vi "Modbus Data Massage New.vi"(10 "register values":u16[](array[numeric]), 11 "Cluster":T1) -> (2 "output cluster":cluster{"Control Name":string, "Value":dbl})   [LabVIEW 2020]
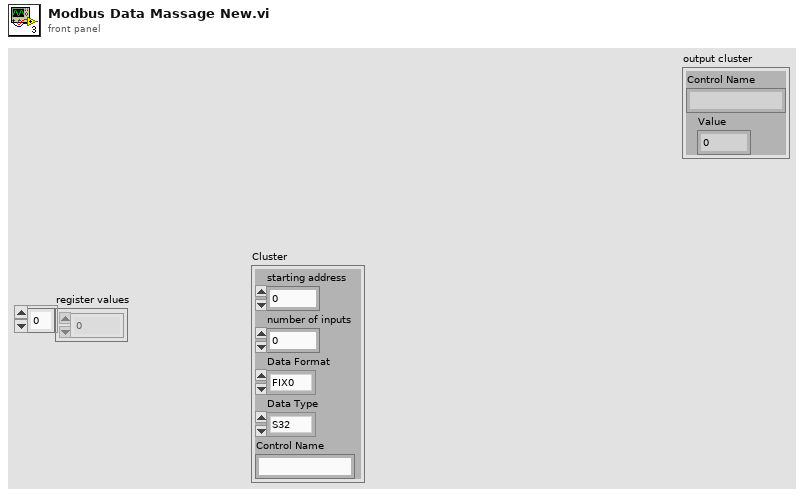
[diagram p1: front panel]
types:
  T1 = cluster{"starting address":u16, "number of inputs":u16, "Data Format":enum16{"FIX0", "FIX1", "FIX2", "FIX3", "FIX4", "FIX5", "FIX6"}, "Data Type":enum16{"S32", "U32", "U64", "S64"}, "Control Name":string}
  T2 = enum16{"FIX0", "FIX1", "FIX2", "FIX3", "FIX4", "FIX5", "FIX6"}
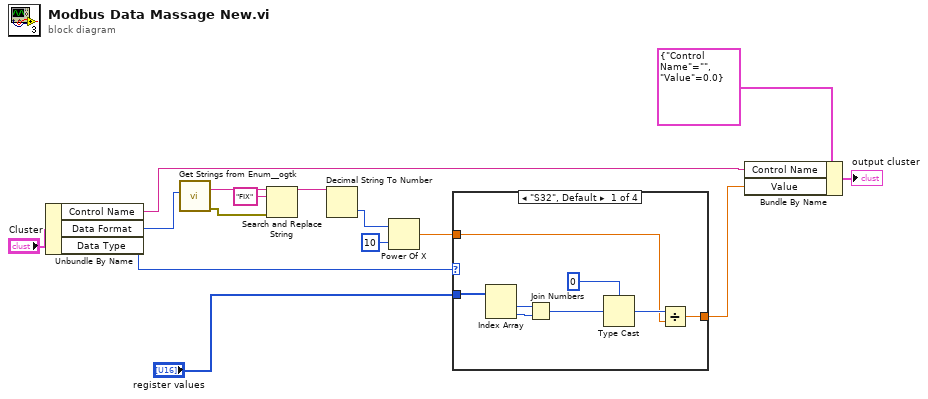
[diagram p0: block diagram]
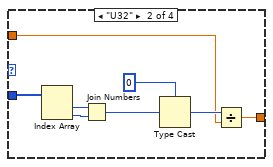
[diagram p2: hidden frame]
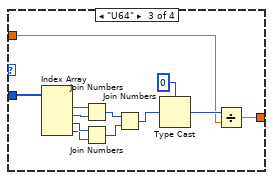
[diagram p3: hidden frame]
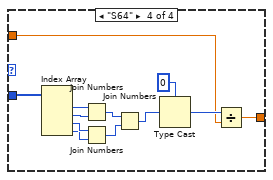
[diagram p4: hidden frame]
diagram:
  n1 = Unbundle By Name("Cluster") -> ("Control Name"=w3:string, "Data Format"=w6:T2, "Data Type"=w13:enum16{"S32", "U32", "U64", "S64"})
  n2 = call <userlib>:"Get Strings from Enum__ogtk.vi"("Enum"=w6) -> ("error out"=w12:errorcluster, "String Value"=w11:string)  [unwired: 7 in, 2 out]
  n3 = Search and Replace String(input string=w11, search string="FIX", error in=w12) -> (result string=w9:string)  [unwired: 5 in, 3 out]
  n4 = Decimal String To Number(string=w9) -> (number=w8:i32)  [unwired: 2 in, 1 out]
  n5 = Power Of X(1:10 ("x"), 2:w8) -> (0:w5:dbl)
  n6 = case shown="\"S32\", Default" w13 {
    tunnel: "register values" -> [w23 w31 w43 w55]
    tunnel: w5 -> [w17 w25 w38 w50]
    tunnel: [w16 w24 w37 w49] -> w2
    frame "S32", Default {
      n7 = Index Array(array=w23) -> (element #1=w22:u16, element #2=w21:u16)  [unwired: 2 in]
      n8 = Join Numbers(hi=w22, lo=w21) -> ((hi.lo)=w20:u32)
      n9 = Type Cast(type=0, x=w20) -> (*(type *) &x=w18:i32)
      n10 = Divide(x=w18, y=w17) -> (x/y=w16:dbl)
    }
    frame "U32" {
      n11 = Index Array(array=w31) -> (element #1=w30:u16, element #2=w29:u16)  [unwired: 2 in]
      n12 = Join Numbers(hi=w30, lo=w29) -> ((hi.lo)=w28:u32)
      n13 = Type Cast(type=u32 0, x=w28) -> (*(type *) &x=w26:u32)
      n14 = Divide(x=w26, y=w25) -> (x/y=w24:dbl)
    }
    frame "U64" {
      n15 = Index Array(array=w43) -> (element #1=w42:u16, element #2=w41:u16, element #3=w36:u16, element #4=w35:u16)  [unwired: 4 in]
      n16 = Join Numbers(hi=w42, lo=w41) -> ((hi.lo)=w34:u32)
      n17 = Join Numbers(hi=w36, lo=w35) -> ((hi.lo)=w33:u32)
      n18 = Join Numbers(hi=w34, lo=w33) -> ((hi.lo)=w32:u64)
      n19 = Type Cast(type=u64 0, x=w32) -> (*(type *) &x=w39:u64)
      n20 = Divide(x=w39, y=w38) -> (x/y=w37:dbl)
    }
    frame "S64" {
      n21 = Index Array(array=w55) -> (element #1=w54:u16, element #2=w53:u16, element #3=w48:u16, element #4=w47:u16)  [unwired: 4 in]
      n22 = Join Numbers(hi=w54, lo=w53) -> ((hi.lo)=w46:u32)
      n23 = Join Numbers(hi=w48, lo=w47) -> ((hi.lo)=w45:u32)
      n24 = Join Numbers(hi=w46, lo=w45) -> ((hi.lo)=w44:u64)
      n25 = Type Cast(type=i64 0, x=w44) -> (*(type *) &x=w51:i64)
      n26 = Divide(x=w51, y=w50) -> (x/y=w49:dbl)
    }
  }
  n27 = Bundle By Name(cluster=cluster{"Control Name":string, "Value":dbl} {"Control Name"="", "Value"=0.0}, "Control Name"=w3, "Value"=w2) -> (→"output cluster":cluster{"Control Name":string, "Value":dbl})
